vi "testPartialCoverage.vi"() -> ()   [LabVIEW 2017, in "CodeCoverageTest.lvlib"]
uses:
  CodeCoverageTest.lvlib
  CodeCoverage/CodeCoverage.lvclass
  Support/Support.lvlib
  33f17cf0-2a6c-41e8-81b1-3bcf142aecf0.vi
panel:
  out "error out":errorcluster
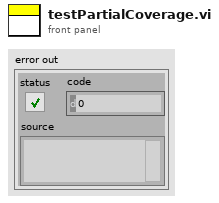
[diagram p1: front panel]
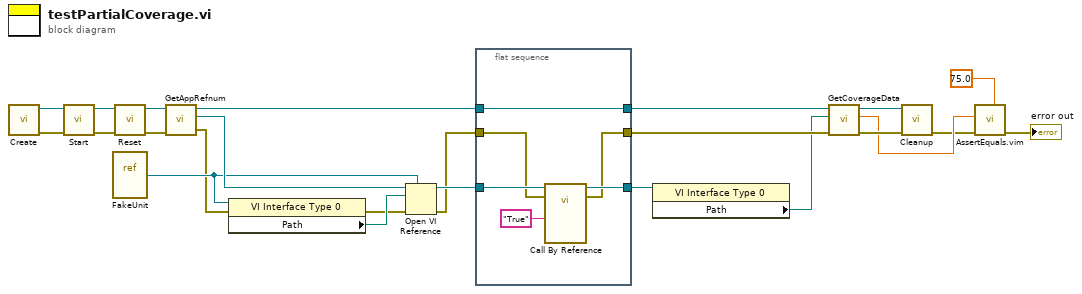
[diagram p0: block diagram]
diagram:
  n1 = call "Create.vi"() -> ("error out"=w23:errorcluster, "CodeCoverage out"=w11:refnum<class "CodeCoverage.lvclass">)  [unwired: 10 in]
  n2 = call "Start.vi"("error in (no error)"=w23, "CodeCoverage in"=w11) -> ("error out"=w17:errorcluster, "CodeCoverage out"=w14:refnum<class "CodeCoverage.lvclass">)  [unwired: 8 in]
  n3 = vi-ref "FakeUnit.vi"() -> (w7:refnum<vi>)
  n4 = call "Reset.vi"("error in (no error)"=w17, "CodeCoverage in"=w14) -> ("error out"=w5:errorcluster, "CodeCoverage out"=w6:refnum<class "CodeCoverage.lvclass">)  [unwired: 8 in]
  n5 = call "GetAppRefnum.vi"("error in (no error)"=w5, "CodeCoverage in"=w6) -> ("error out"=w1:errorcluster, "App Refnum"=w10:refnum<vi>, "CodeCoverage out"=w4:refnum<class "CodeCoverage.lvclass">)  [unwired: 7 in]
  n6 = property class="VI Interface Type 0"(reference=w7, error in=w1) -> (error out=w2:errorcluster, "Path"=w9:path)  [unwired: 1 out]
  n7 = Open VI Reference(type specifier VI Refnum (for type only)=w7, application reference (local)=w10, vi path=w9, error in (no error)=w2) -> (vi reference=w8:refnum<vi>, error out=w3:errorcluster)  [unwired: 2 in]
  n8 = flat-sequence {
    tunnel: [w25] -> w13
    tunnel: w3 -> [w28]
    tunnel: [w26] -> w22
    tunnel: w8 -> [w30]
    tunnel: [w27] -> w21
    tunnel: w4 -> [w25]
    frame #0 {
      n9 = call-by-ref "?"(reference=w30, error in=w28, "Input"="True") -> (reference out=w27:refnum<vi>, error out=w26:errorcluster)  [unwired: 10 in, 1 out]
    }
  }
  n10 = property class="VI Interface Type 0"(reference=w21) -> ("Path"=w20:path)  [unwired: 1 in, 2 out]
  n11 = call "GetCoverageData.vi"("error in (no error)"=w22, "VI Path"=w20, "CodeCoverage in"=w13) -> ("error out"=w24:errorcluster, "Coverage Percentage"=w19:dbl, "CodeCoverage out"=w15:refnum<class "CodeCoverage.lvclass">)  [unwired: 6 in]
  n12 = call "Cleanup.vi"("error in (no error)"=w24, "CodeCoverage in"=w15) -> ("error out"=w16:errorcluster)  [unwired: 9 in]
  n13 = call "AssertEquals.vim"("Expected"=75.0, "error in (no error)"=w16, "Actual"=w19) -> ("error out"=→"error out":errorcluster)  [unwired: 8 in]
